vi "2.3.vi"() -> ()   [LabVIEW 2020]
panel:
  out "Thermometer":dbl(slide) scale=0.0..100.0
  out "Tank":dbl(slide) scale=0.0..10.0
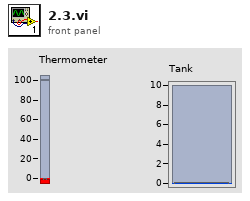
[diagram p1: front panel]
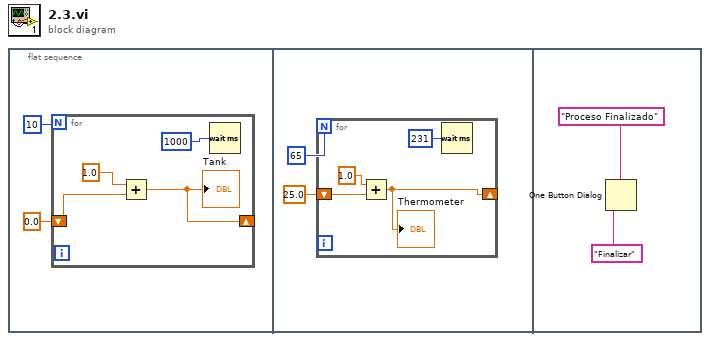
[diagram p0: block diagram]
diagram:
  n1 = flat-sequence {
    frame #0 {
      n2 = for {
        N: 10 -> [_]
        shift-right: [w3] -> _
        shift-left: 0.0 -> [w4]
        n3 = Add(x=1.0, y=w4) -> (x+y=w3:dbl)
        "Tank" <- w3
        n4 = Wait (ms)(milliseconds to wait=u32 1000) -> ()  [unwired: 1 out]
      }
    }
    frame #1 {
      n5 = for {
        N: 65 -> [_]
        shift-right: [w10] -> _
        shift-left: 25.0 -> [w11]
        n6 = Add(x=1.0, y=w11) -> (x+y=w10:dbl)
        "Thermometer" <- w10
        n7 = Wait (ms)(milliseconds to wait=u32 231) -> ()  [unwired: 1 out]
      }
    }
    frame #2 {
      n8 = One Button Dialog(message="Proceso Finalizado", button name ("OK")="Finalizar") -> ()  [unwired: 1 out]
    }
  }
